vi "EnFlo_Tun_Setup_global.vi"() -> ()   [LabVIEW 2018]
panel:
  in  "GDRT DB array":string[][](array[string])
  in  "GDW DB array":string[][](array[string])
  in  "GDE DB array":string[][](array[string])
  in  "Aero Tunnel DB array":string[][](array[string])
  in  "D Tunnel DB array":string[][](array[string])
  in  "A Tunnel DB array":string[][](array[string])
  in  "EnFlo Tun DB array":string[][](array[string])
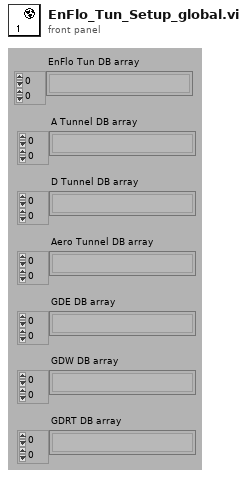
[diagram p1: front panel]
diagram:
